vi "Initialize Configuration File.vi"(8 "error in (no error)":errorcluster, 11 "FP-TC-Shared in":refnum<class "FP-TC-Shared.lvclass">) -> (0 "error out":errorcluster, 2 "Last State Unknown":bool, 3 "FP-TC-Shared out":refnum<class "FP-TC-Shared.lvclass">)   [LabVIEW 2019, in "FP-TC-Shared.lvclass"]
uses:
  FP-TC-Shared.lvclass
  FP-TC-Shared.lvclass/FP-TC-Shared.ctl
  typedefs/LC Type--Enum.ctl
  typedefs/Default PGSQL Paths.ctl
  <userlib>/LevyLab/Instrument Framework/SMOs/Configuration/Configuration.lvclass/Configuration.ctl
  <vilib>/Utility/config.llb/Read Key (String).vi
  <userlib>/LevyLab/Instrument Framework/SMOs/Configuration/Configuration.lvclass
  <vilib>/Utility/config.llb/NI_LVConfig.lvlib
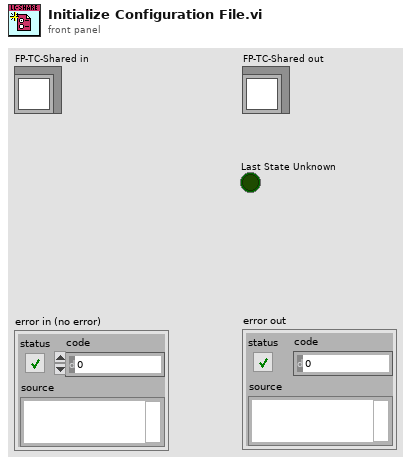
[diagram p1: front panel]
types:
  T1 = typedef "FP-TC-Shared.lvclass/Default PGSQL Paths.ctl" = cluster{"CF.TC":string, "CF.TC.Z":string, "CF.FP":string, "MNK.TC":string, "MNK.TC.Z":string, "MNK.FP":string}
  T2 = typedef "FP-TC-Shared.lvclass/LC Type--Enum.ctl" = enum16{"CF.TC", "CF.TC.Z", "CF.FP", "MNK.TC", "MNK.TC.Z", "MNK.FP"}
  T3 = typedef "NI_LVConfig.lvlib/Config Data RefNum.ctl" = refnum<k1>
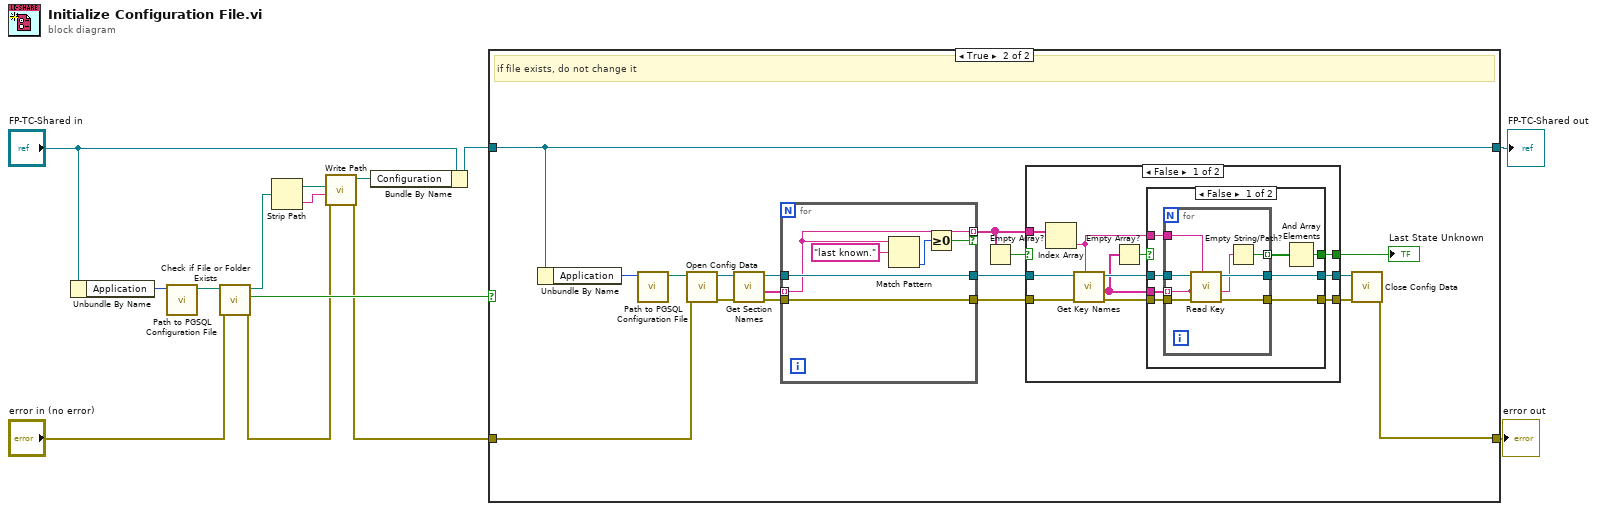
[diagram p0: block diagram]
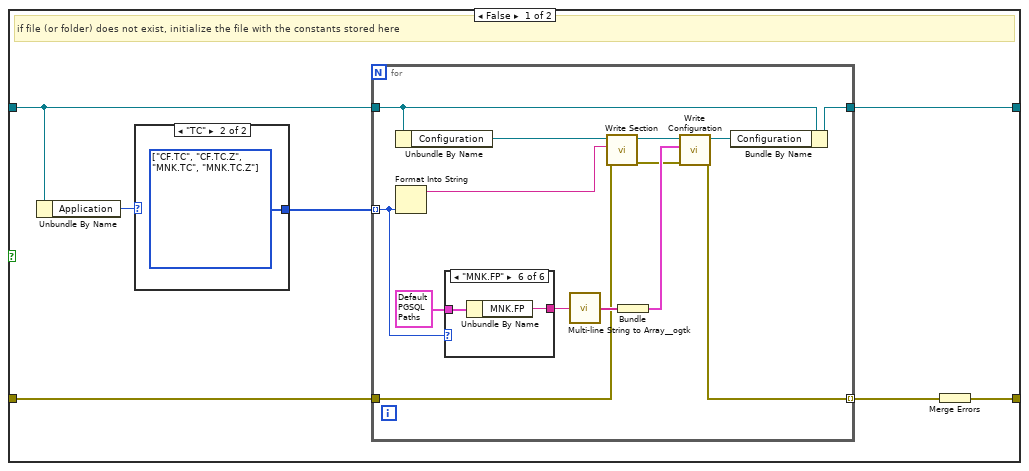
[diagram p2: hidden frame]
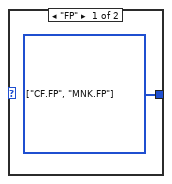
[diagram p3: hidden frame]
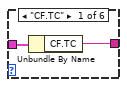
[diagram p4: hidden frame]
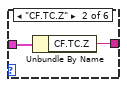
[diagram p5: hidden frame]
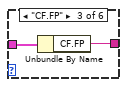
[diagram p6: hidden frame]
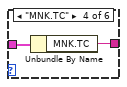
[diagram p7: hidden frame]
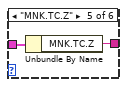
[diagram p8: hidden frame]
diagram:
  n1 = Unbundle By Name("FP-TC-Shared in") -> ("Application"=w10:enum16{"TC", "FP"})
  n2 = call "Path to PGSQL Configuration File.vi"("Application"=w10) -> ("appended path"=w9:path)  [unwired: 10 in]
  n3 = call <vilib>:"Check if File or Folder Exists.vi"("error in (no error)"="error in (no error)", "path"=w9) -> ("error out"=w2:errorcluster, "file or folder exists?"=w11:bool, "dup path"=w7:path)  [unwired: 7 in]
  n4 = Strip Path(path=w7) -> (stripped path=w6:path, name=w8:string)
  n5 = call <userlib>:"Write Path.vi"("error in (no error)"=w2, "Filename [Configuration.ini]"=w8, "Path"=w6) -> ("error out"=w1:errorcluster, "Configuration out"=w3:refnum<class "Configuration.lvclass">)  [unwired: 7 in]
  n6 = Bundle By Name(cluster="FP-TC-Shared in", "Configuration"=w3) -> (w4:refnum<class "FP-TC-Shared.lvclass">)
  n7 = case shown="True" w11 {
    tunnel: [w21 w62] -> w14
    tunnel: w4 -> [w16 w62]
    tunnel: [w19 w50] -> w13
    tunnel: w1 -> [w18 w51]
    frame False {
      # "if file (or folder) does not exist, initialize the file with the constants stored here"
      n8 = Unbundle By Name(w16) -> ("Application"=w15:enum16{"TC", "FP"})
      n9 = case shown="\"TC\"" w15 {
        tunnel: [w22 w23] -> w17
        frame "FP" {
          w22 = T2[] [enum."CF.FP", enum."MNK.FP"] items=["CF.TC", "CF.TC.Z", "CF.FP", "MNK.TC", "MNK.TC.Z", "MNK.FP"] ("Array")
        }
        frame "TC" {
          w23 = T2[] [enum."CF.TC", enum."CF.TC.Z", enum."MNK.TC", enum."MNK.TC.Z"] items=["CF.TC", "CF.TC.Z", "CF.FP", "MNK.TC", "MNK.TC.Z", "MNK.FP"] ("Array")
        }
      }
      n10 = for {
        tunnel: w17 -> [w26] mode=indexing
        tunnel: [w32] -> w21
        tunnel: w18 -> [w28]
        tunnel: w16 -> [w27]
        tunnel: [w34] -> w20 mode=indexing
        n11 = Unbundle By Name(w27) -> ("Configuration"=w24:refnum<class "Configuration.lvclass">)
        n12 = Format Into String(w26) -> (resulting string=w30:string)  [unwired: 3 in, 1 out]
        n13 = case shown="\"MNK.FP\"" w26 {
          tunnel: T1 {"CF.TC"="llab_015:d001(Leiden CF900--CF_TC_R0(ohms))\nllab_015:d002(Leiden CF900--CF_TC_R1(ohms))\nllab_015:d003(Leiden CF900--CF_TC_R2(ohms))\nllab_015:d004(Leiden CF900--CF_TC_R3(ohms))\nllab_015:d005(Leiden CF900--CF_TC_R4(ohms))\nllab_015:d006(Leiden CF900--CF_TC_R5(ohms))\nllab_015:d007(Leiden CF900--CF_TC_R6(ohms))\nllab_015:d008(Leiden CF900--CF_TC_R7(ohms))\nllab_015:d009(Leiden CF900--CF_TC_T0(mK))\nllab_015:d010(Leiden CF900--CF_TC_T1(mK))\nllab_015:d011(Leiden CF900--CF_TC_T2(mK))\nllab_015:d012(Leiden CF900--CF_TC_T3(mK))\nllab_015:d013(Leiden CF900--CF_TC_T4(mK))\nllab_015:d014(Leiden CF900--CF_TC_T5(mK))\nllab_015:d015(Leiden CF900--CF_TC_T6(mK))\nllab_015:d016(Leiden CF900--CF_TC_T7(mK))\nllab_015:d017(Leiden CF900--CF_TC_I0(Amp))\nllab_015:d018(Leiden CF900--CF_TC_I1(Amp))\nllab_015:d019(Leiden CF900--CF_TC_I2(Amp))\nllab_015:d020(Leiden CF900--CF_TC_I3(Amp))\nllab_015:v000(Leiden CF900--CF_TC_description())\nllab_015:v001(Leiden CF900--CF_TC_calibration())", "CF.TC.Z"="llab_015:d021(Leiden CF900--CF_TC_Z_R0(ohms))\nllab_015:d022(Leiden CF900--CF_TC_Z_R1(ohms))\nllab_015:d023(Leiden CF900--CF_TC_Z_R2(ohms))\nllab_015:d024(Leiden CF900--CF_TC_Z_R3(ohms))\nllab_015:d025(Leiden CF900--CF_TC_Z_R4(ohms))\nllab_015:d026(Leiden CF900--CF_TC_Z_R5(ohms))\nllab_015:d027(Leiden CF900--CF_TC_Z_R6(ohms))\nllab_015:d028(Leiden CF900--CF_TC_Z_R7(ohms))\nllab_015:d029(Leiden CF900--CF_TC_Z_R8(ohms))\nllab_015:d030(Leiden CF900--CF_TC_Z_R9(ohms))\nllab_015:d031(Leiden CF900--CF_TC_Z_T0(mK))\nllab_015:d032(Leiden CF900--CF_TC_Z_T1(mK))\nllab_015:d033(Leiden CF900--CF_TC_Z_T2(mK))\nllab_015:d034(Leiden CF900--CF_TC_Z_T3(mK))\nllab_015:d035(Leiden CF900--CF_TC_Z_T4(mK))\nllab_015:d036(Leiden CF900--CF_TC_Z_T5(mK))\nllab_015:d037(Leiden CF900--CF_TC_Z_T6(mK))\nllab_015:d038(Leiden CF900--CF_TC_Z_T7(mK))\nllab_015:d039(Leiden CF900--CF_TC_Z_T8(mK))\nllab_015:d040(Leiden CF900--CF_TC_Z_T9(mK))\nllab_015:v002(Leiden CF900--CF_TC_Z_description())\nllab_015:v003(Leiden CF900--CF_TC_Z_calibration())", "CF.FP"="llab_011:d000(Leiden CF FP--CF_FP_P1(mbar))\nllab_011:d001(Leiden CF FP--CF_FP_P2(mbar))\nllab_011:d002(Leiden CF FP--CF_FP_P3(mbar))\nllab_011:d003(Leiden CF FP--CF_FP_P4(mbar))\nllab_011:d004(Leiden CF FP--CF_FP_P5(mbar))\nllab_011:d005(Leiden CF FP--CF_FP_P6(mbar))\nllab_011:d006(Leiden CF FP--CF_FP_P7(mbar))\nllab_011:d007(Leiden CF FP--CF_FP_Flow())\nllab_011:d008(Leiden CF FP--CF_FP_MG0(mbar))\nllab_011:d009(Leiden CF FP--CF_FP_MG1(mbar))\nllab_011:d010(Leiden CF FP--CF_FP_MG2(mbar))\nllab_011:d011(Leiden CF FP--CF_FP_MG3(mbar))\nllab_011:d012(Leiden CF FP--CF_FP_MG4(mbar))\nllab_011:d013(Leiden CF FP--CF_FP_MG5(mbar))\nllab_011:d014(Leiden CF FP--CF_FP_PT_on())\nllab_011:d015(Leiden CF FP--CF_FP_PT_W_in_T(K))\nllab_011:d016(Leiden CF FP--CF_FP_PT_W_out_T(K))\nllab_011:d017(Leiden CF FP--CF_FP_PT_He_T(K))\nllab_011:d018(Leiden CF FP--CF_FP_PT_oil_T(K))\nllab_011:d019(Leiden CF FP--CF_FP_PT_P_Low(bar))\nllab_011:d020(Leiden CF FP--CF_FP_PT_P_High(bar))\nllab_011:d021(Leiden CF FP--CF_FP_PT_current(A))\nllab_011:d022(Leiden CF FP--CF_FP_state0())\nllab_011:d023(Leiden CF FP--CF_FP_state1())\nllab_011:d024(Leiden CF FP--CF_FP_state2())\nllab_011:v000(Leiden CF FP--CF_FP_STATE())", "MNK.TC"="llab_024:d020(MNK_18T--MNK_TC_R0(ohms))\nllab_024:d039(MNK_18T--MNK_TC_R1(ohms))\nllab_024:d021(MNK_18T--MNK_TC_R2(ohms))\nllab_024:d022(MNK_18T--MNK_TC_R3(ohms))\nllab_024:d037(MNK_18T--MNK_TC_R4(ohms))\nllab_024:d023(MNK_18T--MNK_TC_R5(ohms))\nllab_024:d024(MNK_18T--MNK_TC_R6(ohms))\nllab_024:d025(MNK_18T--MNK_TC_R7(ohms))\nllab_024:d026(MNK_18T--MNK_TC_T0(mK))\nllab_024:d027(MNK_18T--MNK_TC_T1(mK))\nllab_024:d028(MNK_18T--MNK_TC_T2(mK))\nllab_024:d029(MNK_18T--MNK_TC_T3(mK))\nllab_024:d030(MNK_18T--MNK_TC_T4(mK))\nllab_024:d038(MNK_18T--MNK_TC_T5(mK))\nllab_024:d031(MNK_18T--MNK_TC_T6(mK))\nllab_024:d032(MNK_18T--MNK_TC_T7(mK))\nllab_024:d033(MNK_18T--MNK_TC_I0(Amp))\nllab_024:d034(MNK_18T--MNK_TC_I1(Amp))\nllab_024:d035(MNK_18T--MNK_TC_I2(Amp))\nllab_024:d036(MNK_18T--MNK_TC_I3(Amp))\nllab_024:v005(MNK_18T--MNK_TC_description())\nllab_024:v006(MNK_18T--MNK_TC_calibration())", "MNK.TC.Z"="llab_024:d040(MNK_18T--MNK_Cstill_Z(pF))\nllab_024:d041(MNK_18T--MNK_CMN-187_Z(H))\nllab_024:d042(MNK_18T--MNK_Cstill_T(mK))\nllab_024:d043(MNK_18T--MNK_CMN-187_T(mK))\nllab_024:v005(MNK_18T--MNK_TC_Z_description())\nllab_024:v006(MNK_18T--MNK_TC_Z_calibration())", "MNK.FP"="llab_016:d000(Leiden MNK Front Panel--MNK_FP_P1(mbar))\nllab_016:d001(Leiden MNK Front Panel--MNK_FP_P2(mbar))\nllab_016:d002(Leiden MNK Front Panel--MNK_FP_P3(mbar))\nllab_016:d003(Leiden MNK Front Panel--MNK_FP_P4(mbar))\nllab_016:d004(Leiden MNK Front Panel--MNK_FP_P5(mbar))\nllab_016:d005(Leiden MNK Front Panel--MNK_FP_P6(mbar))\nllab_016:d006(Leiden MNK Front Panel--MNK_FP_P7(mbar))\nllab_016:d013(Leiden MNK Front Panel--MNK_FP_Flow())\nllab_016:d007(Leiden MNK Front Panel--MNK_FP_MG0(mbar))\nllab_016:d008(Leiden MNK Front Panel--MNK_FP_MG1(mbar))\nllab_016:d009(Leiden MNK Front Panel--MNK_FP_MG2(mbar))\nllab_016:d010(Leiden MNK Front Panel--MNK_FP_MG3(mbar))\nllab_016:d011(Leiden MNK Front Panel--MNK_FP_MG4(mbar))\nllab_016:d012(Leiden MNK Front Panel--MNK_FP_MG5(mbar))\nllab_016:d014(Leiden MNK Front Panel--MNK_FP_state0())\nllab_016:d015(Leiden MNK Front Panel--MNK_FP_state1())\nllab_016:d016(Leiden MNK Front Panel--MNK_FP_state2())\nllab_016:v000(Leiden MNK Front Panel--MNK_FP_STATE())"} ("PGSQL Paths") -> [w39 w41 w43 w45 w47 w49]
          tunnel: [w38 w40 w42 w44 w46 w48] -> w37
          frame "CF.TC" {
            n14 = Unbundle By Name(w39) -> ("CF.TC"=w38:string)
          }
          frame "CF.TC.Z" {
            n15 = Unbundle By Name(w41) -> ("CF.TC.Z"=w40:string)
          }
          frame "CF.FP" {
            n16 = Unbundle By Name(w43) -> ("CF.FP"=w42:string)
          }
          frame "MNK.TC" {
            n17 = Unbundle By Name(w45) -> ("MNK.TC"=w44:string)
          }
          frame "MNK.TC.Z" {
            n18 = Unbundle By Name(w47) -> ("MNK.TC.Z"=w46:string)
          }
          frame "MNK.FP" {
            n19 = Unbundle By Name(w49) -> ("MNK.FP"=w48:string)
          }
        }
        n20 = call <userlib>:"Multi-line String to Array__ogtk.vi"("string"=w37) -> ("lines"=w36:string[])
        n21 = call <userlib>:"Write Section.vi"("error in (no error)"=w28, "Section"=w30, "Configuration in"=w24) -> ("error out"=w29:errorcluster, "Configuration out"=w31:refnum<class "Configuration.lvclass">)  [unwired: 7 in]
        n22 = Bundle("lines"=w36) -> (w35:cluster{"lines":string[]})  [unwired: 1 in]
        n23 = call <userlib>:"Write Configuration.vi"("error in (no error)"=w29, "Variant"=w35, "Configuration in"=w31) -> ("error out"=w34:errorcluster, "Configuration out"=w25:refnum<class "Configuration.lvclass">)  [unwired: 7 in]
        n24 = Bundle By Name(cluster=w27, "Configuration"=w25) -> (w32:refnum<class "FP-TC-Shared.lvclass">)
      }
      n25 = Merge Errors(w20) -> (w19:errorcluster)
    }
    frame True {
      # "if file exists, do not change it"
      n26 = Unbundle By Name(w62) -> ("Application"=w66:enum16{"TC", "FP"})
      n27 = call "Path to PGSQL Configuration File.vi"("Application"=w66) -> ("appended path"=w65:path)  [unwired: 10 in]
      n28 = call <vilib>:"Open Config Data.vi"("error in (no error)"=w51, "configuration file path"=w65) -> ("error out"=w60:errorcluster, "refnum"=w64:T3)  [unwired: 7 in, 1 out]
      n29 = call <vilib>:"Get Section Names.vi"("error in (no error)"=w60, "refnum"=w64) -> ("error out"=w59:errorcluster, "section names"=w61:string[], "refnum out"=w63:T3)  [unwired: 7 in]
      n30 = for {
        tunnel: w63 -> [w103]
        tunnel: w61 -> [w101] mode=indexing
        tunnel: [w103] -> w57
        tunnel: w59 -> [w102]
        tunnel: [w102] -> w58
        tunnel: [w101] -> w53 mode=indexing if=w100
        n31 = Match Pattern(string=w101, regular expression="last known.") -> (offset past match=w104:i32)  [unwired: 1 in, 3 out]
        n32 = Greater Or Equal To 0?(x=w104) -> (x >= 0?=w100:bool)
      }
      n33 = Empty Array?(array=w53) -> (empty?=w52:bool)
      n34 = case shown="False" w52 {
        selector: w52 -> [_ w97]
        tunnel: w58 -> [w77 w98]
        tunnel: w57 -> [w76 w99]
        tunnel: [w73 w98] -> w56
        tunnel: [w72 w99] -> w55
        tunnel: [w71 w97] -> w54
        tunnel: w53 -> [w70 _]
        frame False {
          n35 = Index Array(array=w70) -> (element=w69:string)  [unwired: 1 in]
          n36 = call <vilib>:"Get Key Names.vi"("section"=w69, "error in (no error)"=w77, "refnum"=w76) -> ("error out"=w74:errorcluster, "key names"=w68:string[], "refnum out"=w75:T3)  [unwired: 5 in, 1 out]
          n37 = Empty Array?(array=w68) -> (empty?=w67:bool)
          n38 = case shown="False" w67 {
            selector: w67 -> [_ w96]
            tunnel: w75 -> [w85 w95]
            tunnel: w74 -> [w84 w94]
            tunnel: [w83 w94] -> w73
            tunnel: [w82 w95] -> w72
            tunnel: [w80 w96] -> w71
            tunnel: w69 -> [w79 _]
            tunnel: w68 -> [w78 _]
            frame False {
              n39 = for {
                tunnel: w85 -> [w93]
                tunnel: [w86] -> _ mode=indexing
                tunnel: w84 -> [w92]
                tunnel: [w91] -> w83
                tunnel: w79 -> [w90]
                tunnel: [w89] -> w82
                tunnel: [w87] -> w81 mode=indexing
                tunnel: w78 -> [w86] mode=indexing
                n40 = call-poly <vilib>:"Read Key.vi"("section"=w90, "error in (no error)"=w92, "key"=w86, "refnum"=w93) -> ("error out"=w91:errorcluster, "value"=w88:string, "refnum out"=w89:T3)  [unwired: 4 in, 1 out]
                n41 = Empty String/Path?(string/path=w88) -> (empty?=w87:bool)
              }
              n42 = And Array Elements(Boolean array=w81) -> (logical AND=w80:bool)
            }
            frame True {
            }
          }
        }
        frame True {
        }
      }
      "Last State Unknown" <- w54
      n43 = call <vilib>:"Close Config Data.vi"("error in (no error)"=w56, "refnum"=w55) -> ("error out"=w50:errorcluster)  [unwired: 8 in, 1 out]
    }
  }
  "FP-TC-Shared out" <- w14
  "error out" <- w13
